vi "Read IG and CG Pressure.vi"(8 "error in (no error)":errorcluster, 11 "VISA resource name":refnum<visa-resource-name>="COM7") -> (0 "error out":errorcluster, 3 "Data":dbl[](array[numeric]))   [LabVIEW 2022 SP3, in "Lesker Pressure.lvclass"]
uses:
  Lesker Pressure.lvclass
  Lesker Pressure.lvclass/Lesker Pressure.ctl
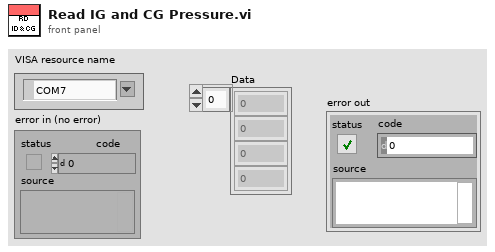
[diagram p1: front panel]
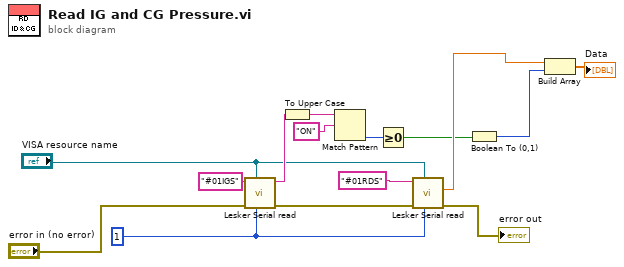
[diagram p0: block diagram]
diagram:
  w6 = 1 ("Number of reads")
  n1 = call "Lesker Serial read.vi"("Number of reads"=w6, "VISA resource name"="VISA resource name", "error in (no error)"="error in (no error)", "Command"="#01IGS") -> ("error out"=w7:errorcluster, "Response"=w14:string)  [unwired: 5 in, 1 out]
  n2 = To Upper Case(1:w14) -> (0:w10:string)
  n3 = Match Pattern(string=w10, regular expression="ON") -> (offset past match=w12:i32)  [unwired: 1 in, 3 out]
  n4 = Greater Or Equal To 0?(x=w12) -> (x >= 0?=w2:bool)
  n5 = call "Lesker Serial read.vi"("Number of reads"=w6, "VISA resource name"="VISA resource name", "error in (no error)"=w7, "Command"="#01RDS") -> ("error out"=→"error out":errorcluster, "Pressure"=w3:dbl)  [unwired: 5 in, 1 out]
  n6 = Boolean To (0,1)(Boolean=w2) -> (0, 1=w11:i16)
  n7 = Build Array(w3, w11) -> (→"Data":dbl[])
